vi "RPC Method Register.vi"(8 "error in (no error)":errorcluster, 11 "OOP Server in":refnum<class "Query Server.lvclass">) -> (0 "error out":errorcluster, 3 "OOP Server out":refnum<class "Query Server.lvclass">)   [LabVIEW 2016, in "Query Server.lvlib" / "Query Server.lvclass"]
uses:
  Query Server.lvclass
  gRPC lvSupport/Server API/typeDefs/grpcId.ctl
  gRPC lvSupport/gprc-lvsupport.lvlib
  RPC Messages/ServerEvent/ServerEvent_Data.ctl
  typeDefs/Server State Data.ctl
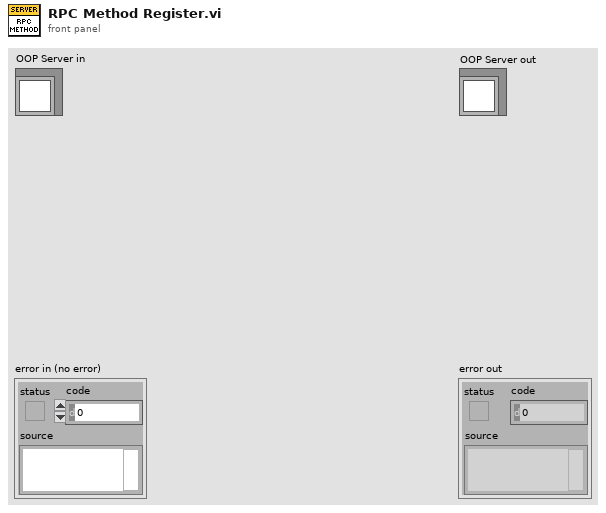
[diagram p1: front panel]
types:
  T1 = typedef "Query Server.lvlib/gprc-lvsupport.lvlib/grpcId.ctl" = u64
  T2 = typedef "Query Server.lvlib/Query Server.lvclass/Server State Data.ctl" = cluster{"Data":string}
  T3 = typedef "Query Server.lvlib/Query Server.lvclass/ServerEvent_Data.ctl" = cluster{"eventData":string, "serverId":i32, "status":i32}
  T4 = typedef "Query Server.lvlib/Query Server.lvclass/Server Internal UEs.ctl" = cluster{"Invoke Internal UE":refnum<user-event>, "Query Internal UE":refnum<user-event>, "Register Internal UE":refnum<user-event>}
  T5 = typedef "Query Server.lvlib/Query Server.lvclass/Server gRPC UEs.ctl" = cluster{"Invoke gRPC UE":refnum<user-event>, "Query gRPC UE":refnum<user-event>, "Register gRPC UE":refnum<user-event>}
  T6 = typedef "Query Server.lvlib/Query Server.lvclass/RegistrationRequest_Data.ctl" = cluster{"eventName":string}
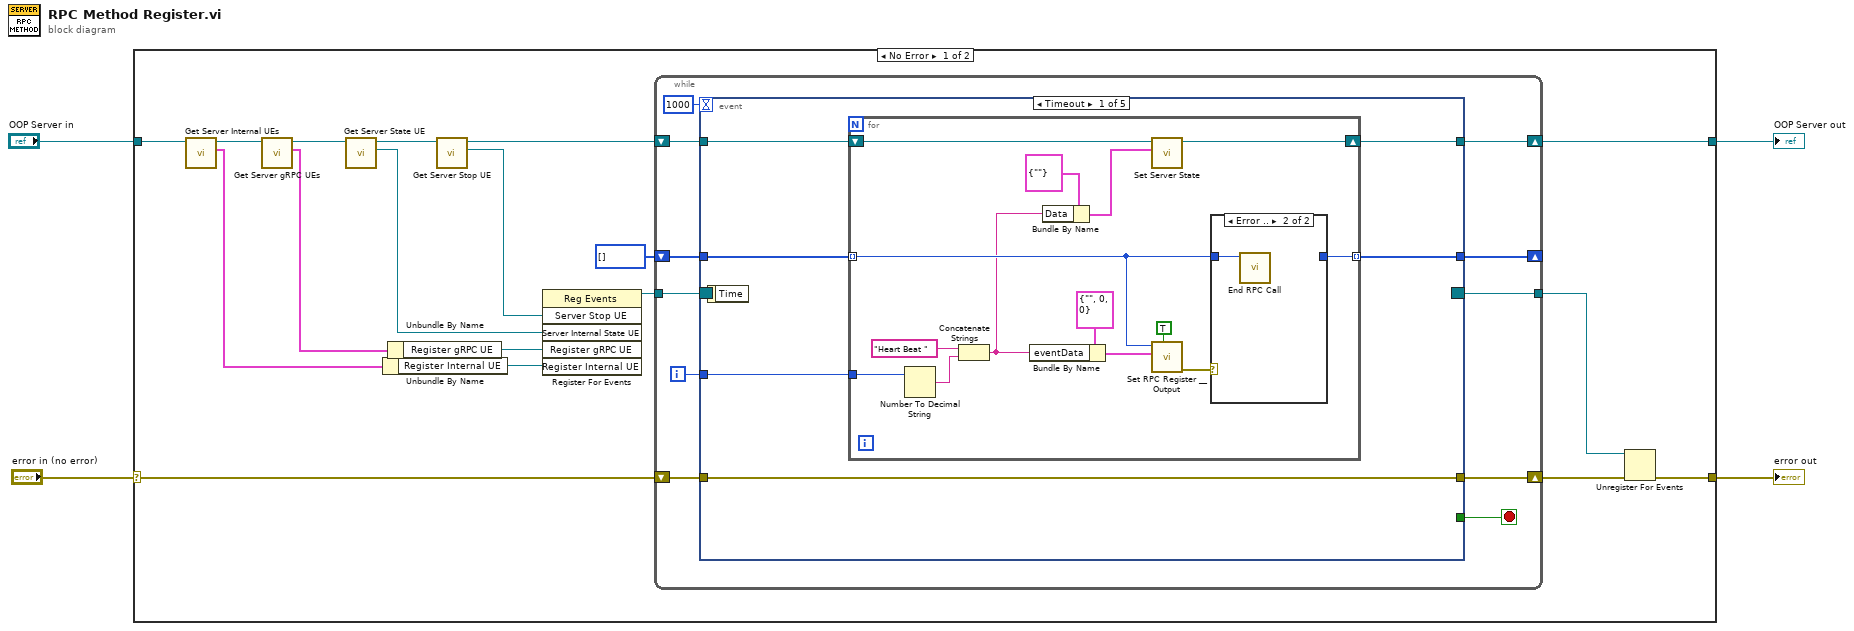
[diagram p0: block diagram]
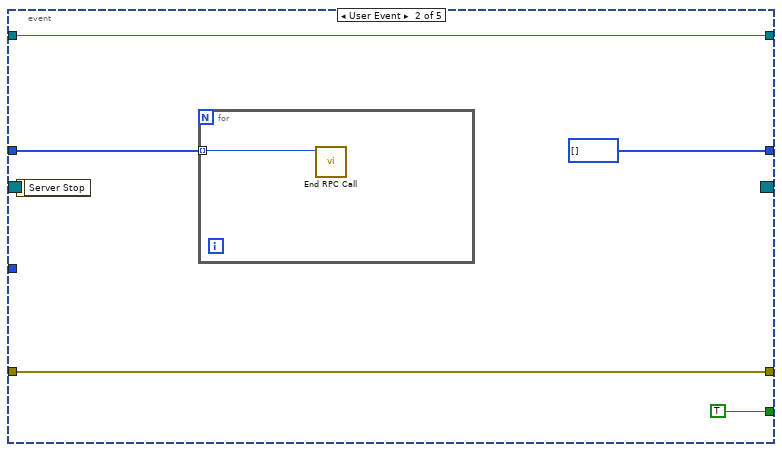
[diagram p3: hidden frame]
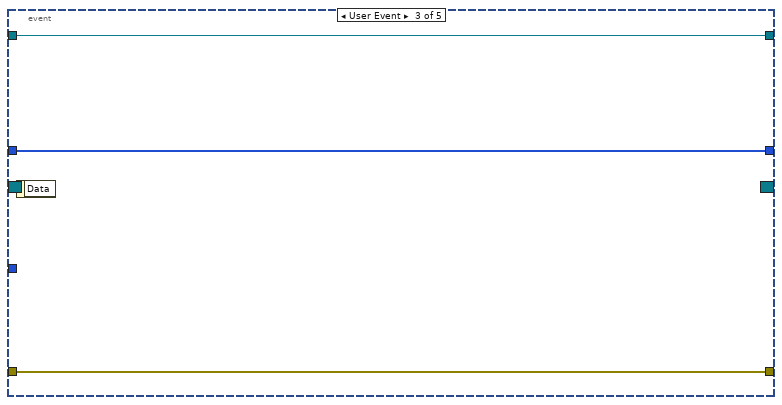
[diagram p4: hidden frame]
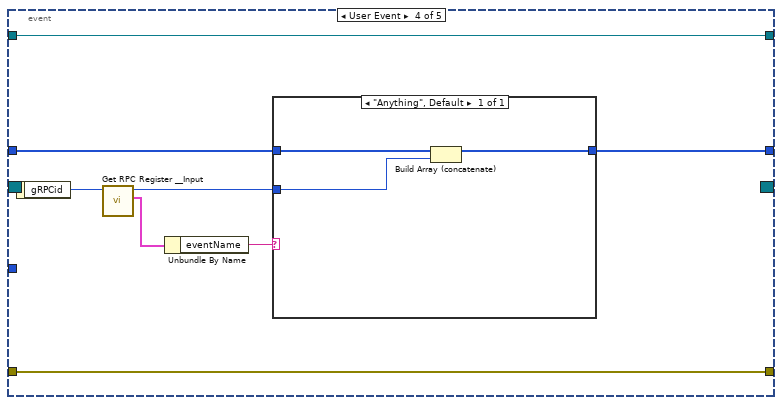
[diagram p5: hidden frame]
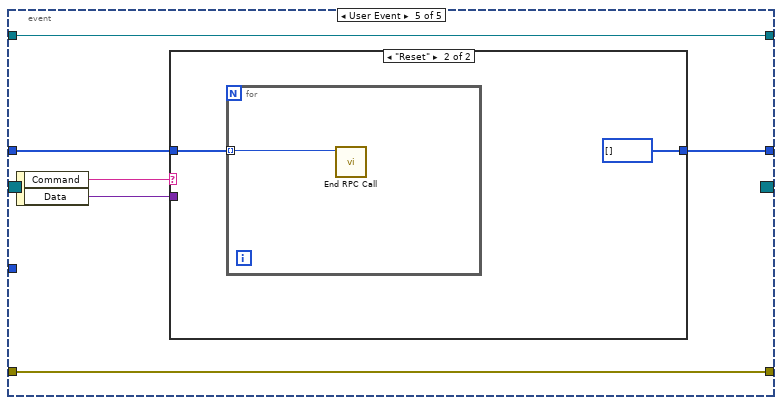
[diagram p6: hidden frame]
diagram:
  n1 = case shown="No Error" "error in (no error)" {
    selector: "error in (no error)" -> [w18 w87]
    tunnel: [w16 w87] -> w3
    tunnel: "OOP Server in" -> [w20 w86]
    tunnel: [w6 w86] -> w1
    frame No Error {
      n2 = call "Get Server Internal UEs.vi"("OOP Server in"=w20) -> ("Server Internal UEs"=w12:T4, "OOP Server out"=w19:refnum<class "Query Server.lvclass">)  [unwired: 9 in]
      n3 = call "Get Server gRPC UEs.vi"("OOP Server in"=w19) -> ("Server gRPC UEs"=w14:T5, "OOP Server out"=w9:refnum<class "Query Server.lvclass">)  [unwired: 8 in, 1 out]
      n4 = call "Get Server State UE.vi"("Template Server in"=w9) -> ("Server Internal State UE"=w7:refnum<user-event>, "Template Server out"=w8:refnum<class "Query Server.lvclass">)  [unwired: 9 in]
      n5 = Unbundle By Name ("Unbundle Internal UE")(w12) -> ("Register Internal UE"=w11:refnum<user-event>)
      n6 = Unbundle By Name ("Unbundle gRPC UE")(w14) -> ("Register gRPC UE"=w13:refnum<user-event>)
      n7 = call "Get Server Stop UE.vi"("OOP Server in"=w8) -> ("Server Stop UE"=w22:refnum<user-event>, "OOP Server out"=w10:refnum<class "Query Server.lvclass">)  [unwired: 9 in]
      n8 = register-events(w22, w7, w13, w11) -> (reference out=w21:refnum<event-registration>)  [unwired: 2 in, 1 out]
      n9 = while {
        tunnel: w21 -> [w33]
        tunnel: [w29] -> w15
        shift-right: [w30] -> w17
        shift-left: w18 -> [w31]
        shift-right: [w27] -> w6
        shift-left: w10 -> [w28]
        shift-right: [w26] -> _
        shift-left: T1[] [] -> [w25]
        i -> [w24]
        stop <- w32 stop-if-true
        n10 = event "RPC Method Event Structure" shown="[0] Timeout" {
          selector: w33 -> [_ _ _ _ _]
          dyn-events: [_ _ _ _ _] -> w29
          timeout: 1000 -> [_ _ _ _ _]
          tunnel: [_ TRUE _ _ _] -> w32
          tunnel: w31 -> [w39 w59 w64 w72 w81]
          tunnel: [w39 w59 w64 w72 w81] -> w30
          tunnel: w28 -> [w35 w58 w63 w71 w80]
          tunnel: [w34 w58 w63 w71 w80] -> w27
          tunnel: [w36 T1[] [] w62 w66 w76] -> w26
          tunnel: w25 -> [w38 w57 w62 w65 w77]
          tunnel: w24 -> [w37 _ _ _ _]
          event Timeout {
            n11 = event-data() -> ()  [unwired: 1 in, 1 out]
            n12 = for {
              tunnel: w38 -> [w47] mode=indexing
              tunnel: w37 -> [w51]
              tunnel: [w46] -> w36 mode=indexing
              shift-right: [w44] -> w34
              shift-left: w35 -> [w45]
              n13 = Number To Decimal String(number=w51) -> (decimal integer string=w53:string)  [unwired: 1 in]
              n14 = Concatenate Strings("Heart Beat " ("eventdata"), w53) -> (w41:string)
              n15 = Bundle By Name(cluster=T3 {"eventData"="", "serverId"=0, "status"=0} ("Message Data"), "eventData"=w41) -> (w49:T3)
              n16 = Bundle By Name(cluster=T2 {"Data"=""} ("New State"), "Data"=w41) -> (w42:T2)
              n17 = call "Set Server State.vi"("New State"=w42, "Template Server in"=w45) -> ("Template Server out"=w44:refnum<class "Query Server.lvclass">)  [unwired: 7 in, 2 out]
              n18 = call "Set RPC Register __Output.vi"("Streeming? (F)"=TRUE, "Message Data"=w49, "gRPCid in"=w47) -> ("error out"=w48:errorcluster)  [unwired: 8 in]
              n19 = case shown="Error .." w48 {
                tunnel: w47 -> [w54 w55]
                tunnel: [w54 _] -> w46
                frame No Error {
                }
                frame Error {
                  n20 = call "End RPC Call.vi"("gRPCid"=w55) -> ()  [unwired: 10 in, 1 out]
                }
              }
            }
          }
          event User Event {
            n21 = event-data() -> ()  [unwired: 1 in, 1 out]
            n22 = for {
              tunnel: w57 -> [w61] mode=indexing
              n23 = call "End RPC Call.vi"("gRPCid"=w61) -> ()  [unwired: 10 in, 1 out]
            }
          }
          event User Event {
            n24 = event-data() -> ()  [unwired: 1 in, 1 out]
          }
          event User Event {
            n25 = event-data() -> ("gRPCid"=w70:T1)  [unwired: 1 in]
            n26 = call "Get RPC Register __Input.vi"("gRPCid in"=w70) -> ("Message Data"=w69:T6, "gRPCid out"=w67:T1)  [unwired: 8 in, 1 out]
            n27 = Unbundle By Name(w69) -> ("eventName"=w68:string)
            n28 = case shown="\"Anything\", Default" w68 {
              tunnel: w67 -> [w75]
              tunnel: [w74] -> w66
              tunnel: w65 -> [w73]
              frame "Anything", Default {
                n29 = Build Array (concatenate)(w73, w75) -> (w74:T1[])
              }
            }
          }
          event User Event {
            n30 = event-data() -> ("Command"=w79:string, "Data"=w78:variant)  [unwired: 1 in]
            n31 = case shown="\"Reset\"" w79 {
              tunnel: w78 -> [_ _]
              tunnel: w77 -> [w82 w84]
              tunnel: [w82 T1[] []] -> w76
              frame "None", Default {
              }
              frame "Reset" {
                n32 = for {
                  tunnel: w84 -> [w85] mode=indexing
                  n33 = call "End RPC Call.vi"("gRPCid"=w85) -> ()  [unwired: 10 in, 1 out]
                }
              }
            }
          }
        }
      }
      n34 = Unregister For Events(event registration refnum=w15, error in=w17) -> (error out=w16:errorcluster)
    }
    frame Error {
    }
  }
  "error out" <- w3
  "OOP Server out" <- w1
